vi "Write Naming Data.vi"(8 "error in":errorcluster, 10 "Approval Tests.lvlib:Naming Data.lvclass":refnum<class "Naming Data.lvclass">, 11 "Options in":refnum<class "Options.lvclass">) -> (0 "error out":errorcluster, 3 "Options out":refnum<class "Options.lvclass">)   [LabVIEW 2020, in "Approval Tests.lvlib" / "Options.lvclass"]
uses:
  Options.lvclass
  Naming Data/Naming Data.lvclass
  Options.lvclass/Options.ctl
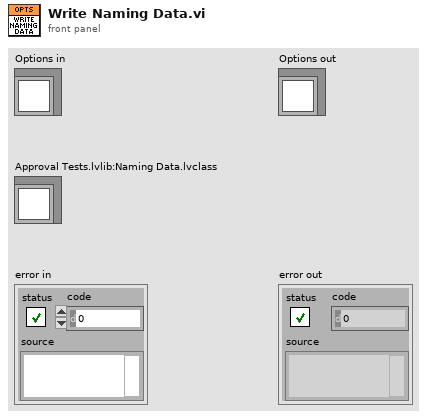
[diagram p1: front panel]
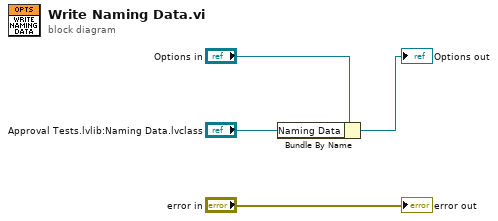
[diagram p0: block diagram]
diagram:
  n1 = Bundle By Name(cluster="Options in", "Naming Data"="Approval Tests.lvlib:Naming Data.lvclass") -> (→"Options out":refnum<class "Options.lvclass">)
  "error out" <- "error in"
